vi "Center.vi"(0 "FSM.Graph In":refnum<class "FSM.Graph.lvclass">, 7 "Draw Area Size":T1) -> (4 "FSM.Graph Out":refnum<class "FSM.Graph.lvclass">)   [LabVIEW 2020, in "FSM.Graph.lvclass"]
uses:
  FSM.Graph.lvclass
  <vilib>/Utility/miscctls.llb/LVBoundsTypeDef.ctl
  FSM.Graph.lvclass/FSM.Graph.ctl
  FSM.Node/FSM.Node.lvclass/FSM.Node.ctl
  FSM.Edge/FSM.Edge.lvclass/FSM.Edge.ctl
  FSM.Node/Read rect.vi
  FSM.Edge/Read Points.vi
  FSM.Node/FSM.Node.lvclass
  FSM.Edge/FSM.Edge.lvclass
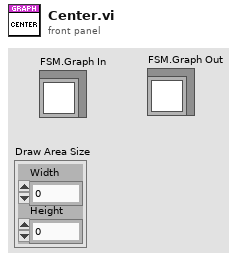
[diagram p1: front panel]
types:
  T1 = typedef "LVBoundsTypeDef.ctl" = cluster{"Width":u32, "Height":u32}
  T2 = cluster{"left":i16, "top":i16, "right":i16, "bottom":i16}
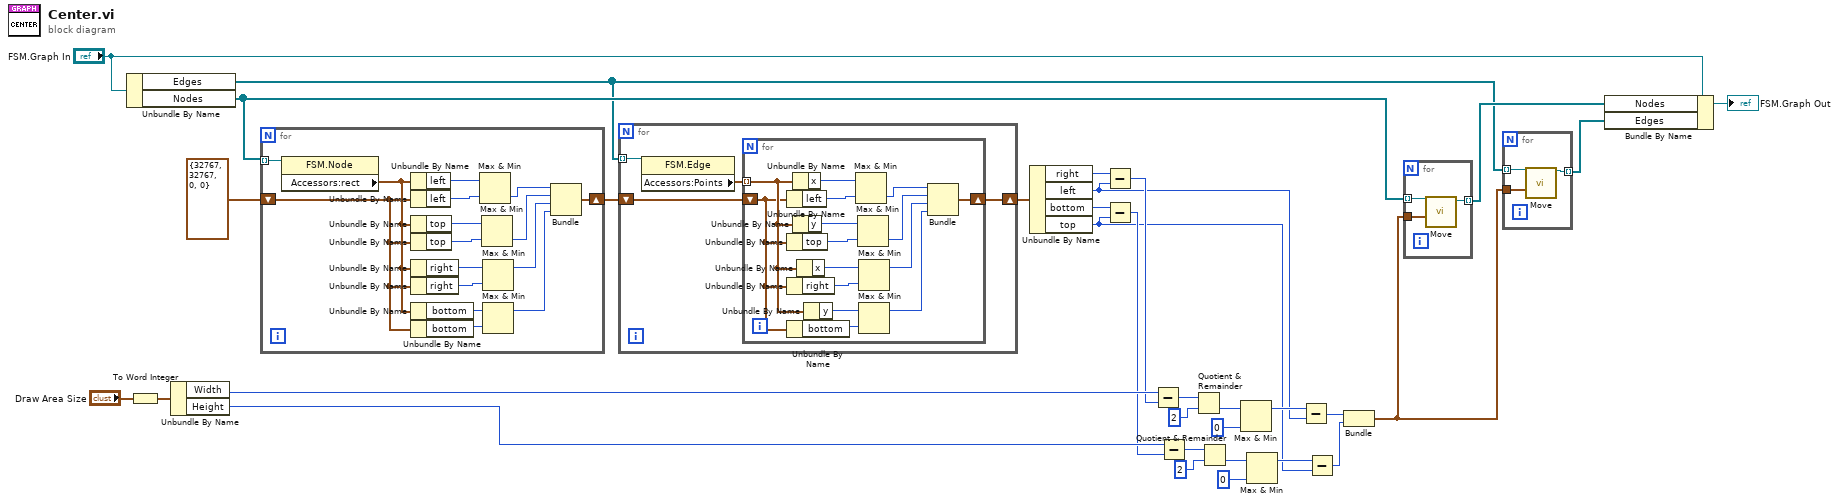
[diagram p0: block diagram]
diagram:
  n1 = Unbundle By Name("FSM.Graph In") -> ("Edges"=w1:refnum<class "FSM.Edge.lvclass">[], "Nodes"=w21:refnum<class "FSM.Node.lvclass">[])
  n2 = To Word Integer(number="Draw Area Size") -> (16bit integer=w6:cluster{"Width":i16, "Height":i16})
  n3 = Unbundle By Name(w6) -> ("Width"=w29:i16, "Height"=w12:i16)
  n4 = for {
    tunnel: w21 -> [w48] mode=indexing
    shift-right: [w38] -> w3
    shift-left: T2 {"left"=32767, "top"=32767, "right"=0, "bottom"=0} ("rect") -> [w33]
    n5 = property class="FSM.Node"(reference=w48) -> ("Accessors:rect"=w39:T2)  [unwired: 1 in, 2 out]
    n6 = Unbundle By Name(w39) -> ("left"=w47:i16)
    n7 = Unbundle By Name(w33) -> ("left"=w46:i16)
    n8 = Unbundle By Name(w39) -> ("top"=w45:i16)
    n9 = Unbundle By Name(w33) -> ("top"=w44:i16)
    n10 = Unbundle By Name(w39) -> ("right"=w43:i16)
    n11 = Unbundle By Name(w33) -> ("right"=w42:i16)
    n12 = Unbundle By Name(w39) -> ("bottom"=w41:i16)
    n13 = Unbundle By Name(w33) -> ("bottom"=w40:i16)
    n14 = Max & Min(x=w47, y=w46) -> (min(x,y)=w37:i16)  [unwired: 1 out]
    n15 = Max & Min(x=w45, y=w44) -> (min(x,y)=w36:i16)  [unwired: 1 out]
    n16 = Max & Min(x=w43, y=w42) -> (max(x,y)=w35:i16)  [unwired: 1 out]
    n17 = Max & Min(x=w41, y=w40) -> (max(x,y)=w34:i16)  [unwired: 1 out]
    n18 = Bundle(w37, w36, w35, w34) -> (w38:cluster{i16, i16, i16, i16})  [unwired: 1 in]
  }
  n19 = for {
    tunnel: w1 -> [w52] mode=indexing
    shift-right: [w50] -> w2
    shift-left: w3 -> [w49]
    n20 = property class="FSM.Edge"(reference=w52) -> ("Accessors:Points"=w51:cluster{"x":i16, "y":i16}[])  [unwired: 1 in, 2 out]
    n21 = for {
      tunnel: w51 -> [w59] mode=indexing
      shift-right: [w58] -> w50
      shift-left: w49 -> [w53]
      n22 = Unbundle By Name(w53) -> ("left"=w66:i16)
      n23 = Unbundle By Name(w53) -> ("top"=w64:i16)
      n24 = Unbundle By Name(w53) -> ("right"=w62:i16)
      n25 = Unbundle By Name(w53) -> ("bottom"=w60:i16)
      n26 = Unbundle By Name(w59) -> ("x"=w67:i16)
      n27 = Unbundle By Name(w59) -> ("y"=w65:i16)
      n28 = Unbundle By Name(w59) -> ("x"=w63:i16)
      n29 = Unbundle By Name(w59) -> ("y"=w61:i16)
      n30 = Max & Min(x=w67, y=w66) -> (min(x,y)=w57:i16)  [unwired: 1 out]
      n31 = Max & Min(x=w65, y=w64) -> (min(x,y)=w56:i16)  [unwired: 1 out]
      n32 = Max & Min(x=w63, y=w62) -> (max(x,y)=w55:i16)  [unwired: 1 out]
      n33 = Max & Min(x=w61, y=w60) -> (max(x,y)=w54:i16)  [unwired: 1 out]
      n34 = Bundle(w57, w56, w55, w54) -> (w58:cluster{i16, i16, i16, i16})  [unwired: 1 in]
    }
  }
  n35 = Unbundle By Name(w2) -> ("right"=w22:i16, "left"=w5:i16, "bottom"=w10:i16, "top"=w4:i16)
  n36 = Subtract(x=w22, y=w5) -> (x-y=w28:i16)
  n37 = Subtract(x=w10, y=w4) -> (x-y=w11:i16)
  n38 = Subtract(x=w29, y=w28) -> (x-y=w27:i16)
  n39 = Subtract(x=w12, y=w11) -> (x-y=w17:i16)
  n40 = Quotient & Remainder(x=w27, y=2) -> (floor(x/y)=w25:i32)  [unwired: 1 out]
  n41 = Quotient & Remainder(x=w17, y=2) -> (floor(x/y)=w15:i32)  [unwired: 1 out]
  n42 = Max & Min(x=w25, y=0) -> (max(x,y)=w23:i32)  [unwired: 1 out]
  n43 = Max & Min(x=w15, y=0) -> (max(x,y)=w13:i32)  [unwired: 1 out]
  n44 = Subtract(x=w23, y=w5) -> (x-y=w18:i32)
  n45 = Subtract(x=w13, y=w4) -> (x-y=w9:i32)
  n46 = Bundle(w18, w9) -> (w8:cluster{i32, i32})  [unwired: 1 in]
  n47 = for {
    tunnel: w21 -> [w70] mode=indexing
    tunnel: [w69] -> w19 mode=indexing
    tunnel: w8 -> [w68]
    n48 = call "Move.vi"("delta"=w68, "FSM in"=w70) -> ("FSM out"=w69:refnum<class "FSM.Node.lvclass">)  [unwired: 8 in, 1 out]
  }
  n49 = for {
    tunnel: w1 -> [w73] mode=indexing
    tunnel: [w72] -> w7 mode=indexing
    tunnel: w8 -> [w71]
    n50 = call "Move.vi"("FSM.Edge in"=w73, "delta"=w71) -> ("FSM.Edge out"=w72:refnum<class "FSM.Edge.lvclass">)  [unwired: 13 in]
  }
  n51 = Bundle By Name(cluster="FSM.Graph In", "Nodes"=w19, "Edges"=w7) -> (→"FSM.Graph Out":refnum<class "FSM.Graph.lvclass">)
